vi "Test Amplitude Class.vi"(8 "error in (no error)":errorcluster, 11 "TestCase in":refnum<class "Test FGEN.lvclass">) -> (0 "error out":errorcluster, 3 "TestCase out":refnum<class "Test FGEN.lvclass">)   [LabVIEW 2020, in "Test FGEN.lvclass"]
uses:
  Test FGEN.lvclass
  Libraries/FGen/Generador/Generador.lvclass
  Libraries/FGen/GeneradorAmplificado/GeneradorAmplificado.lvclass
  C:/Users/scrap/Fork/IVIsaac2P/IVIsaac2Parcial/Libraries/FGen/Generador/Generador.lvclass
  <vilib>/measure/mascope.llb/Amplitude and Levels 1 chan.vi
  <vilib>/addons/_JKI Toolkits/VI Tester/TestCase.llb/TestCase.lvclass
  <vilib>/measure/NI_MAPro.lvlib
  C:/Program Files (x86)/National Instruments/LabVIEW 2020/vi.lib/addons/_JKI Toolkits/VI Tester/TestCase.llb/TestCase.lvclass
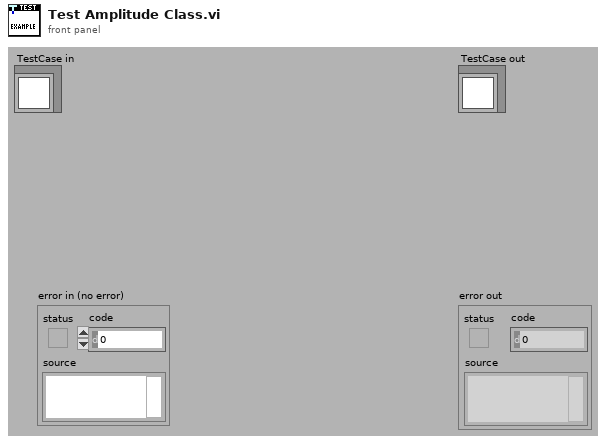
[diagram p1: front panel]
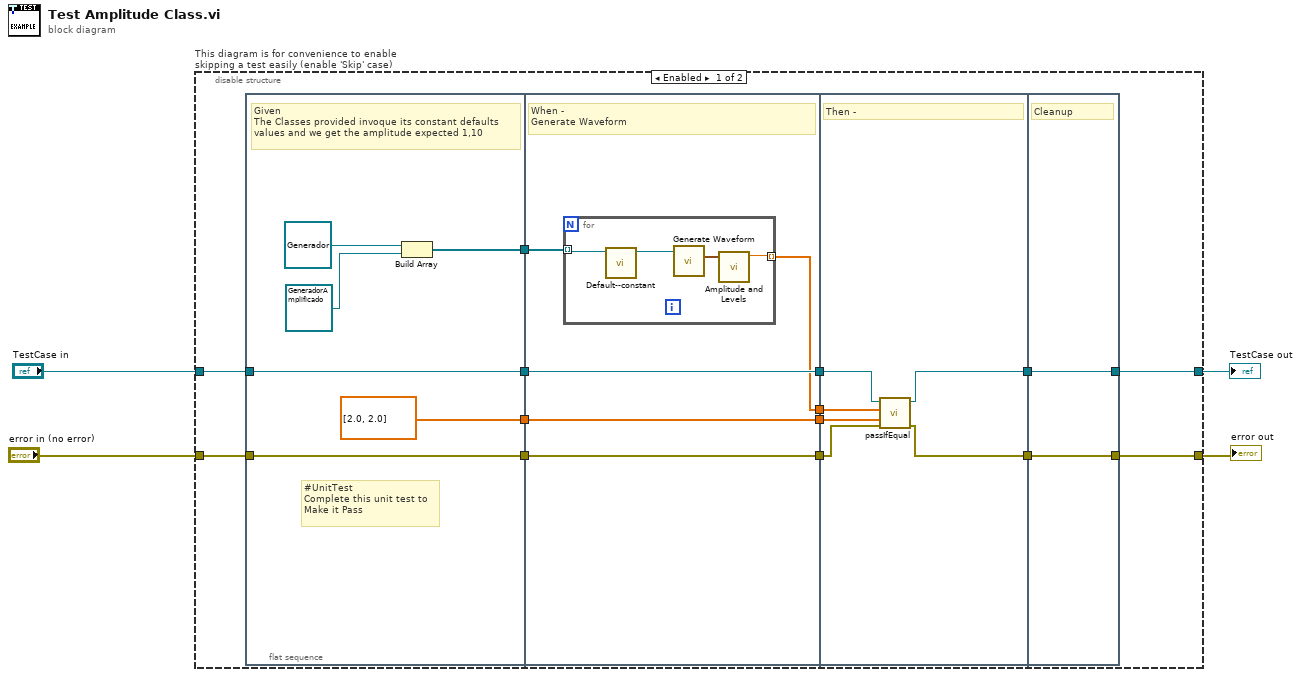
[diagram p0: block diagram]
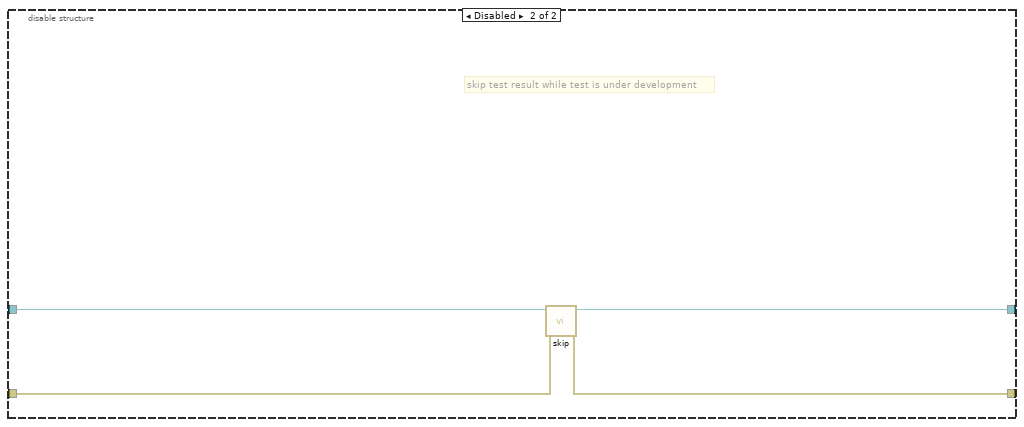
[diagram p2: hidden frame]
diagram:
  n1 = disable-structure "This diagram is for convenience to enable skipping a test easily (enable 'Skip' case)" shown="Enabled" {
    disable-tunnel: "TestCase in" -> [w14 w45]
    disable-tunnel: [w12 w43] -> w1
    disable-tunnel: [w13 w44] -> w3
    disable-tunnel: "error in (no error)" -> [w11 w42]
    frame Enabled {
      n2 = flat-sequence {
        tunnel: w14 -> [w24]
        tunnel: [w24] -> w18
        tunnel: w11 -> [w23]
        tunnel: [w23] -> w9
        tunnel: [dbl[] [2.0, 2.0]] -> w7
        tunnel: [w19] -> w5
        tunnel: [w29] -> w17
        tunnel: w18 -> [w29]
        tunnel: [w28] -> w10
        tunnel: w9 -> [w28]
        tunnel: [w27] -> w8
        tunnel: w7 -> [w26]
        tunnel: [w26] -> w6
        tunnel: w5 -> [w25]
        tunnel: [w38] -> w16
        tunnel: [w37] -> w15
        tunnel: w17 -> [w39]
        tunnel: w10 -> [w36]
        tunnel: w8 -> [w35]
        tunnel: w6 -> [w34]
        tunnel: [w40] -> w13
        tunnel: [w41] -> w12
        tunnel: w16 -> [w41]
        tunnel: w15 -> [w40]
        frame #0 {
          # "#UnitTest\nComplete this unit test to\nMake it Pass"
          # "Given\nThe Classes provided invoque its constant defaults values and we get the amplitude expected 1,10"
          n3 = Build Array(refnum<class "Generador.lvclass"> refnum ("FGen.lvlib:Generator"), refnum<class "GeneradorAmplificado.lvclass"> refnum ("FGen.lvlib:GeneradorAmplificado.lvclass")) -> (w19:refnum<class "Generador.lvclass">[])
        }
        frame #1 {
          # "When -\nGenerate Waveform"
          n4 = for {
            tunnel: [w33] -> w27 mode=indexing
            tunnel: w25 -> [w30] mode=indexing
            n5 = call-dynamic "Default--constant.vi"("Generator in"=w30) -> ("Generator out"=w31:refnum<class "Generador.lvclass">)  [unwired: 9 in, 1 out]
            n6 = call "Generate Waveform.vi"("Generator in"=w31) -> ("Waveform"=w32:waveform(dbl))  [unwired: 8 in, 2 out]
            n7 = call-poly <vilib>:"Amplitude and Levels.vi"("signal in"=w32) -> ("amplitude"=w33:dbl)  [unwired: 7 in, 3 out]
          }
        }
        frame #2 {
          # "Then -"
          n8 = call-dynamic "passIfEqual.vi"("error in (no error)"=w36, "y"=w34, "x"=w35, "TestCase in"=w39) -> ("error out"=w37:errorcluster, "TestCase out"=w38:refnum<class "Test FGEN.lvclass">)  [unwired: 6 in]
        }
        frame #3 {
          # "Cleanup"
        }
      }
    }
    frame Disabled {
      # "skip test result while test is under development"
      n9 = call <vilib>:"skip.vi"("error in (no error)"=w42, "TestCase in"=w45) -> ("error out"=w44:errorcluster, "TestCase out"=w43:refnum<class "Test FGEN.lvclass">)  [unwired: 8 in]
    }
  }
  "error out" <- w3
  "TestCase out" <- w1
